vi "InitHH_AnyThread.vi"(9 "mode":T2 items=["Histo"=0, "T2"=2, "T3"=3, "Conti"=8], 10 "refsource":T3, 11 "Library Version":string="3.0") -> (0 "error out":errorcluster, 2 "Init Info":T1, 3 "DevIdx":i32)   [LabVIEW 2017]
uses:
  HH_RefSource.ctl
  HH_MeasMode.ctl
  HH_InitInfo.ctl
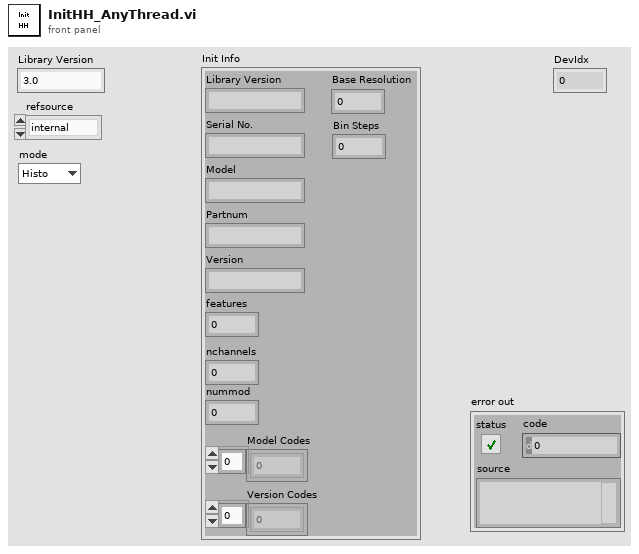
[diagram p1: front panel]
types:
  T1 = typedef "HH_InitInfo.ctl" = cluster{"Library Version":string, "Serial No.":string, "Model":string, "Partnum":string, "Version":string, "features":i32, "nchannels":i32, "nummod":i32, "Model Codes":i32[], "Version Codes":i32[], "Base Resolution":dbl, "Bin Steps":i32}
  T2 = typedef "HH_MeasMode.ctl" = i32
  T3 = typedef "HH_RefSource.ctl" = enum16{"internal", "external"}
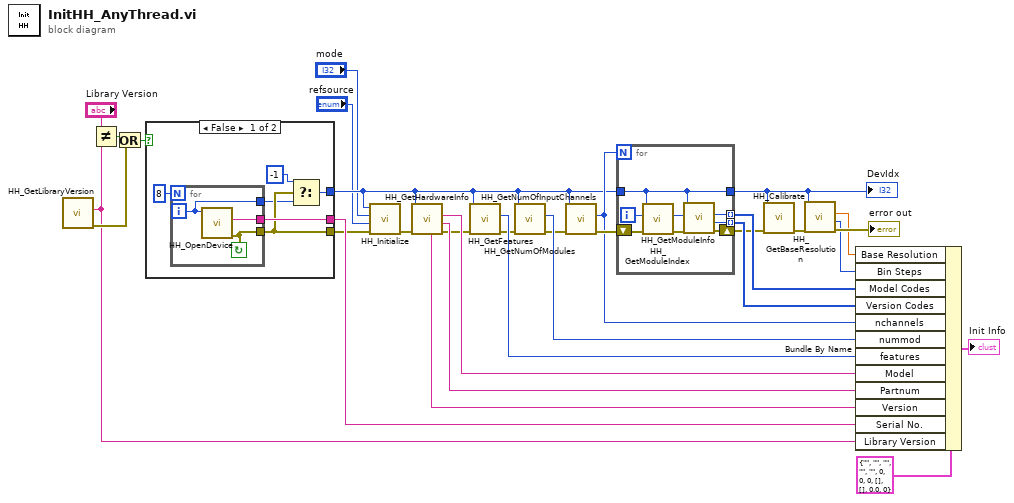
[diagram p0: block diagram]
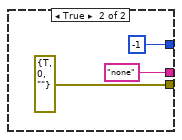
[diagram p2: hidden frame]
diagram:
  n1 = call "HH_GetLibraryVersion.vi"() -> ("error out"=w30:errorcluster, "Version"=w20:string)  [unwired: 9 in, 1 out]
  n2 = Not Equal?(x="Library Version", y=w20) -> (x != y?=w29:bool)
  n3 = Or(x=w29, y=w30) -> (x .or. y?=w28:bool)
  n4 = case shown="False" w28 {
    tunnel: [w33 -1 ("return type")] -> w4
    tunnel: [w36 "none" ("serial")] -> w22
    tunnel: [w35 errorcluster {"status"=TRUE, "code"=0, "source"=""} ("error out")] -> w1
    frame False {
      n5 = for {
        N: 8 -> [_]
        tunnel: [w39] -> w35
        tunnel: [w38] -> w36
        tunnel: [w40] -> w34
        i -> [w40]
        stop <- w39 continue-if-true
        n6 = call "HH_OpenDevice.vi"("devidx"=w40) -> ("error out"=w39:errorcluster, "serial"=w38:string)  [unwired: 8 in, 1 out]
      }
      n7 = Select(t=-1, s=w35, f=w34) -> (s? t:f=w33:i32)
    }
    frame True {
    }
  }
  n8 = call "HH_Initialize.vi"("error in (no error)"=w1, "refsource"="refsource", "mode"="mode", "devidx"=w4) -> ("error out"=w27:errorcluster)  [unwired: 6 in, 1 out]
  n9 = call "HH_GetHardwareInfo.vi"("error in (no error)"=w27, "devidx"=w4) -> ("error out"=w18:errorcluster, "Partnum"=w25:string, "Model"=w26:string, "Version"=w24:string)  [unwired: 5 in, 1 out]
  n10 = call "HH_GetFeatures.vi"("error in (no error)"=w18, "devidx"=w4) -> ("error out"=w17:errorcluster, "features"=w23:i32)  [unwired: 7 in, 1 out]
  n11 = call "HH_GetNumOfModules.vi"("error in (no error)"=w17, "devidx"=w4) -> ("error out"=w15:errorcluster, "nummod"=w16:i32)  [unwired: 7 in, 1 out]
  n12 = call "HH_GetNumOfInputChannels.vi"("error in (no error)"=w15, "devidx"=w4) -> ("error out"=w14:errorcluster, "nchannels"=w13:i32)  [unwired: 7 in, 1 out]
  n13 = for {
    N: w13 -> [_]
    tunnel: w4 -> [w45]
    tunnel: [w48] -> w12 mode=indexing
    tunnel: [w47] -> w11 mode=indexing
    tunnel: [w45] -> w8
    shift-right: [w44] -> w10
    shift-left: w14 -> [w51]
    i -> [w46]
    n14 = call "HH_GetModuleIndex.vi"("error in (no error)"=w51, "channel"=w46, "devidx"=w45) -> ("error out"=w49:errorcluster, "modidx"=w50:i32)  [unwired: 6 in, 1 out]
    n15 = call "HH_GetModuleInfo.vi"("error in (no error)"=w49, "modidx"=w50, "devidx"=w45) -> ("error out"=w44:errorcluster, "versioncode"=w48:i32, "modelcode"=w47:i32)  [unwired: 5 in, 1 out]
  }
  "DevIdx" <- w8
  n16 = call "HH_Calibrate.vi"("error in (no error)"=w10, "devidx"=w8) -> ("error out"=w9:errorcluster)  [unwired: 8 in, 1 out]
  n17 = call "HH_GetBaseResolution.vi"("error in (no error)"=w9, "devidx"=w8) -> ("error out"=→"error out":errorcluster, "binsteps"=w6:i32, "resolution"=w5:dbl)  [unwired: 6 in, 1 out]
  n18 = Bundle By Name(cluster=T1 {"Library Version"="", "Serial No."="", "Model"="", "Partnum"="", "Version"="", "features"=0, "nchannels"=0, "nummod"=0, "Model Codes"=[], "Version Codes"=[], "Base Resolution"=0.0, "Bin Steps"=0} ("Init"), "Base Resolution"=w5, "Bin Steps"=w6, "Model Codes"=w11, "Version Codes"=w12, "nchannels"=w13, "nummod"=w16, "features"=w23, "Model"=w26, "Partnum"=w25, "Version"=w24, "Serial No."=w22, "Library Version"=w20) -> (→"Init Info":T1)
